vi "Display_Anzeige_Select.vi"(6 "X/Y/W/H":i32[](array[numeric]), 7 "Decider":i32[](array[numeric]), 8 "error in (no error)":errorcluster, 9 "Decision":bool, 11 "VISA Refnum in":refnum<visa-resource-name>) -> (0 "error out":errorcluster, 3 "VISA Refnum out":refnum<visa-resource-name>)   [LabVIEW 2018]
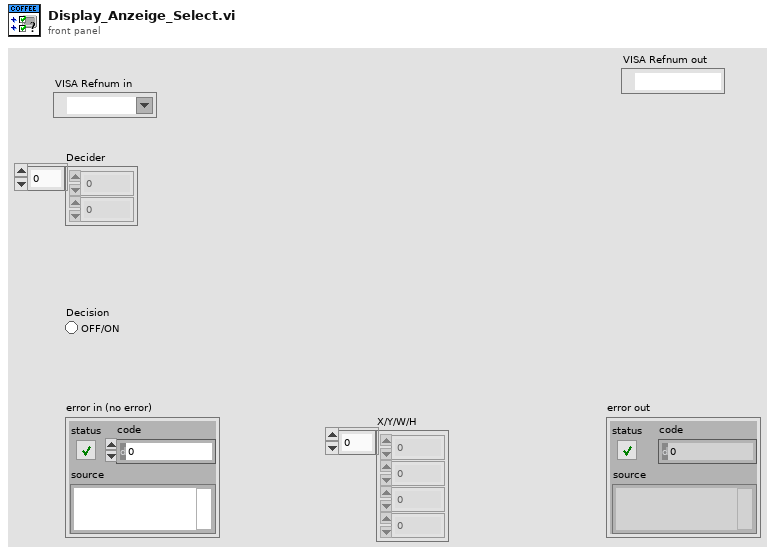
[diagram p1: front panel]
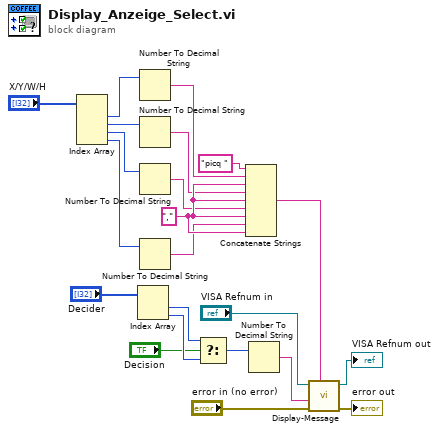
[diagram p0: block diagram]
diagram:
  w15 = ","
  n1 = Index Array(array="X/Y/W/H") -> (element #1=w20:i32, element #2=w19:i32, element #3=w18:i32, element #4=w17:i32)  [unwired: 4 in]
  n2 = Index Array(array="Decider") -> (element #1=w4:i32, element #2=w3:i32)  [unwired: 2 in]
  n3 = Number To Decimal String(number=w20) -> (decimal integer string=w16:string)  [unwired: 1 in]
  n4 = Number To Decimal String(number=w19) -> (decimal integer string=w14:string)  [unwired: 1 in]
  n5 = Number To Decimal String(number=w18) -> (decimal integer string=w13:string)  [unwired: 1 in]
  n6 = Number To Decimal String(number=w17) -> (decimal integer string=w12:string)  [unwired: 1 in]
  n7 = Select(t=w4, s="Decision", f=w3) -> (s? t:f=w6:i32)
  n8 = Concatenate Strings("picq ", w16, w15, w14, w15, w13, w15, w12, w15) -> (w11:string)
  n9 = Number To Decimal String(number=w6) -> (decimal integer string=w2:string)  [unwired: 1 in]
  n10 = call "Display-Message.vi"("Element"=w11, "error in (no error)"="error in (no error)", "Message"=w2, "VISA Refnum in"="VISA Refnum in") -> ("error out"=→"error out":errorcluster, "VISA Refnum out"=→"VISA Refnum out":refnum<visa-resource-name>)  [unwired: 6 in]
